vi "加标回收参数设置.vi"() -> ()   [LabVIEW 2016, in "质控单元V4.lvlib"]
panel:
  in  "布尔":bool
  in  "Tab Control 2":enum32{"氨氮", "总磷", "总氮", "高锰酸盐指数", "化学需氧量"}(tab)
  out "氨氮加标回收率":sgl caption="加标回收率" format="%#.2f"
  out "氨氮加标体积":sgl caption="加标体积" format="%#.4f"
  in  "氨氮母液浓度":sgl caption="母液浓度"
  in  "氨氮定容体积":sgl caption="定容体积"
  out "氨氮加标后水样浓度":sgl caption="加标后水样浓度" format="%#.4f"
  out "氨氮加标前水样浓度":sgl caption="加标前水样浓度" format="%#.4f"
  in  "氨氮量程":sgl caption="量程"
  in  "氨氮检出限":sgl caption="检出限"
  out "TP加标回收率":sgl caption="加标回收率" format="%#.2f"
  out "TP加标体积":sgl caption="加标体积" format="%#.4f"
  in  "TP母液浓度":sgl caption="母液浓度"
  in  "TP定容体积":sgl caption="定容体积"
  out "TP加标后水样浓度":sgl caption="加标后水样浓度" format="%#.4f"
  out "TP加标前水样浓度":sgl caption="加标前水样浓度" format="%#.4g"
  in  "TP量程":sgl caption="量程"
  in  "TP检出限":sgl caption="检出限"
  out "TN加标回收率":sgl caption="加标回收率" format="%#.2f"
  out "TN加标体积":sgl caption="加标体积" format="%#.4f"
  in  "TN母液浓度":sgl caption="母液浓度"
  in  "TN定容体积":sgl caption="定容体积"
  out "TN加标后水样浓度":sgl caption="加标后水样浓度" format="%#.4f"
  out "TN加标前水样浓度":sgl caption="加标前水样浓度" format="%#.4f"
  in  "TN量程":sgl caption="量程"
  in  "TN检出限":sgl caption="检出限"
  out "CODMn加标回收率":sgl caption="加标回收率" format="%#.2f"
  out "CODMn加标体积":sgl caption="加标体积" format="%#.4f"
  in  "CODMn母液浓度":sgl caption="母液浓度"
  in  "CODMn定容体积":sgl caption="定容体积"
  out "CODMn加标后水样浓度":sgl caption="加标后水样浓度" format="%#.4f"
  out "CODMn加标前水样浓度":sgl caption="加标前水样浓度" format="%#.4f"
  in  "CODMn量程":sgl caption="量程"
  in  "CODMn检出限":sgl caption="检出限"
  out "CODCr加标回收率":sgl caption="加标回收率" format="%#.2f"
  out "CODCr加标体积":sgl caption="加标体积" format="%#.4f"
  in  "CODCr母液浓度":sgl caption="母液浓度"
  in  "CODCr定容体积":sgl caption="定容体积"
  out "CODCr加标后水样浓度":sgl caption="加标后水样浓度" format="%#.4f"
  out "CODCr加标前水样浓度":sgl caption="加标前水样浓度" format="%#.4f"
  in  "CODCr量程":sgl caption="量程"
  in  "CODCr检出限":sgl caption="检出限"
  # "加标回收参数设置"
  # "加标回收参数"
  # "加标回收参数"
  # "加标回收参数"
  # "加标回收参数"
  # "加标回收参数"
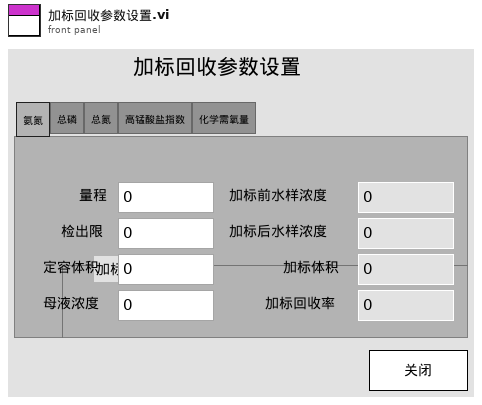
[diagram p1: front panel]
types:
  T1 = cluster{"量程":dbl, "检出限":dbl, "加标前水样浓度":dbl, "加标后水样浓度":dbl, "加标水杯定容体积":dbl, "加标母液浓度":dbl, "加标体积":dbl, "加标回收率":dbl}
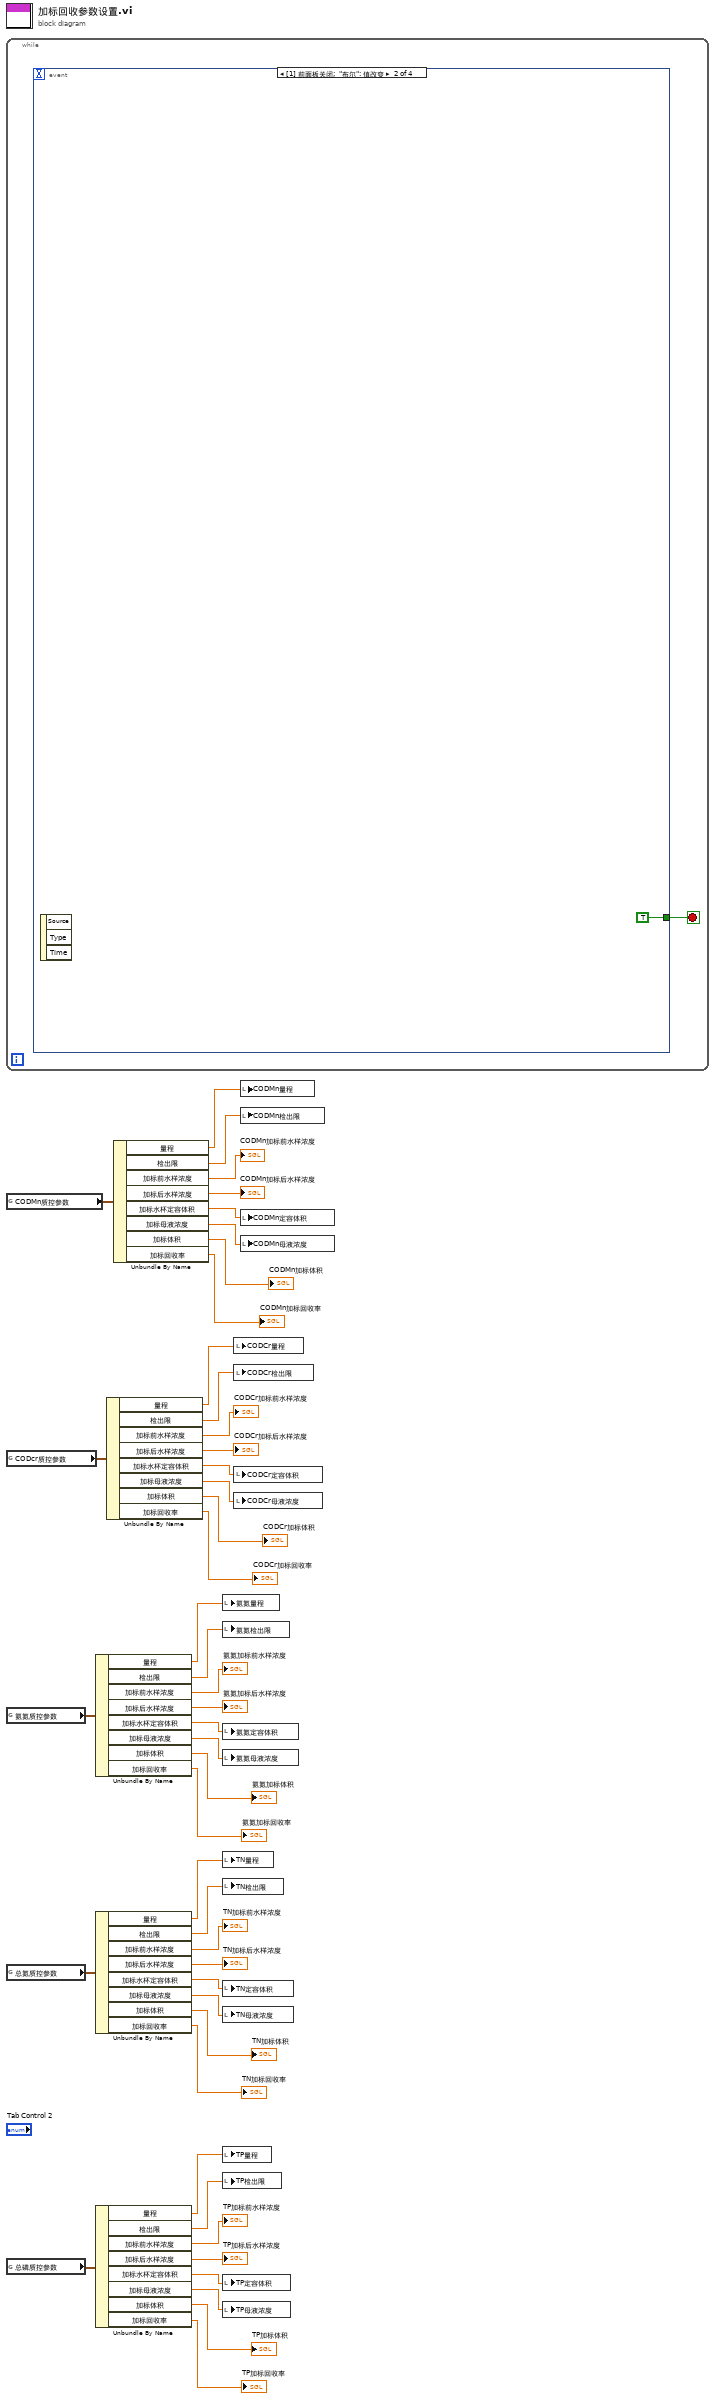
[diagram p0: block diagram]
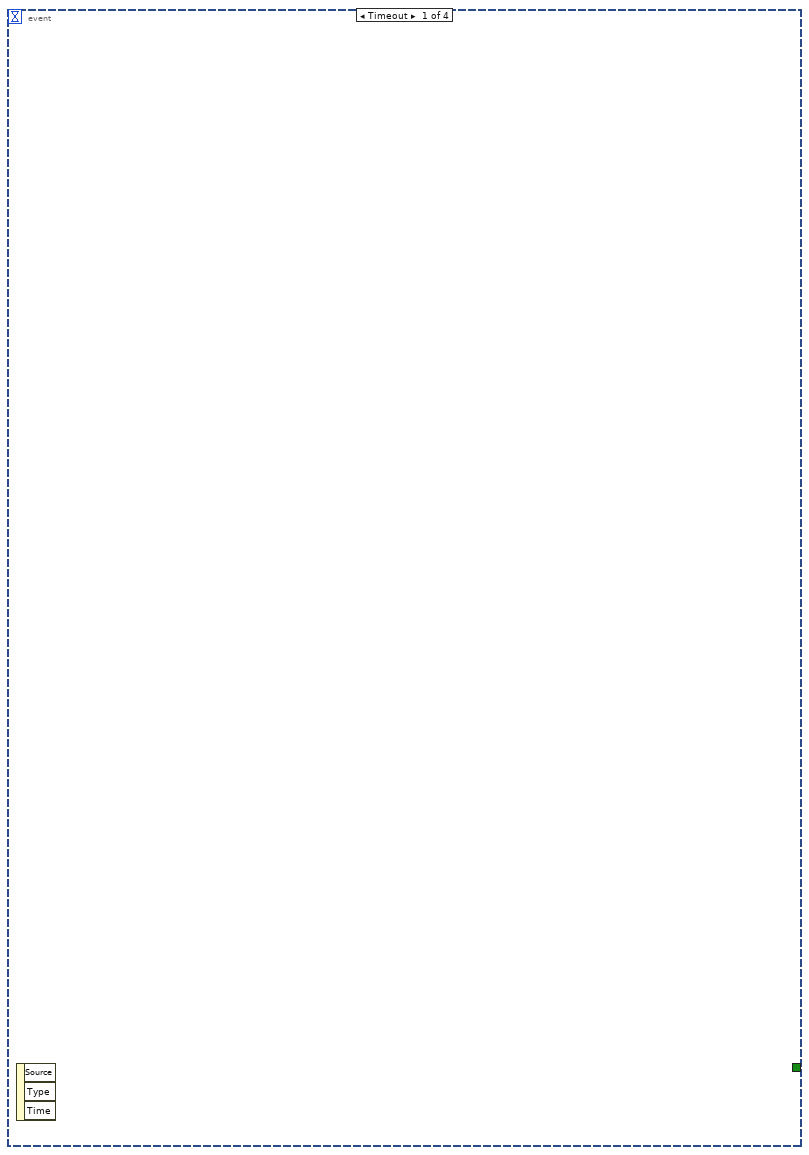
[diagram p2: hidden frame]
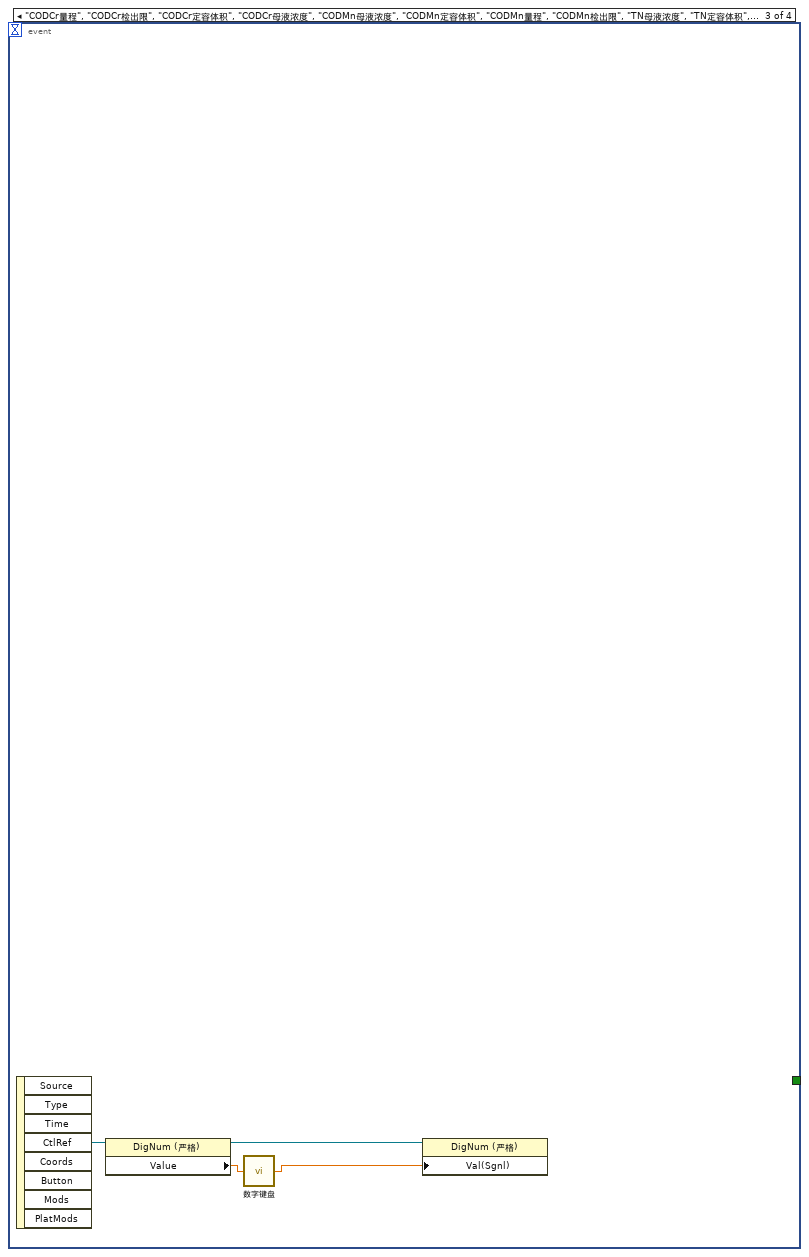
[diagram p3: hidden frame]
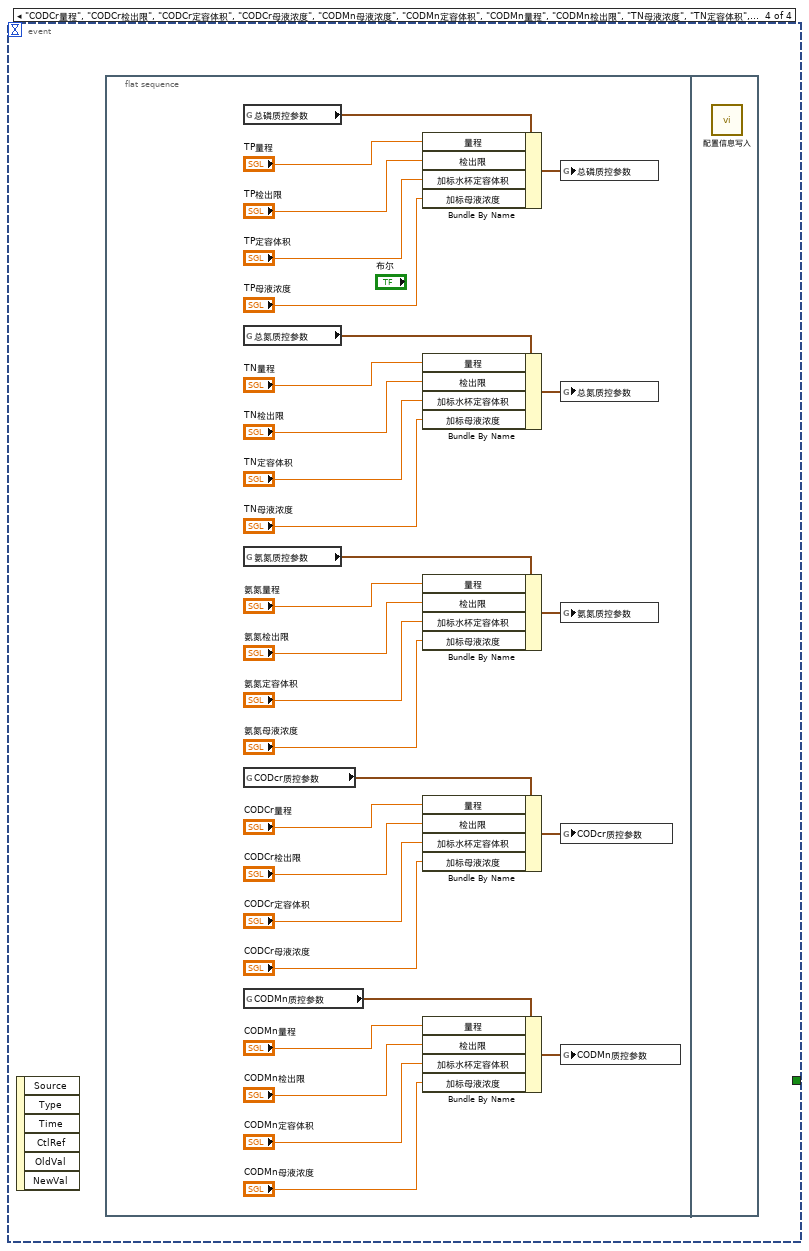
[diagram p4: hidden frame]
diagram:
  n1 = while {
    stop <- w46 stop-if-true
    n2 = event shown="[1] 前面板关闭;  \"布尔\": 值改变" {
      selector: _ -> [_ _ _ _]
      dyn-events: _ -> [_ _ _ _]
      timeout: _ -> [_ _ _ _]
      tunnel: [_ TRUE _ _] -> w46
      event Timeout {
        n3 = event-data() -> ()  [unwired: 1 in, 3 out]
      }
      event Panel Close; "布尔": Value Change {
        n4 = event-data() -> ()  [unwired: 1 in, 3 out]
      }
      event "CODCr量程", "CODCr检出限", "CODCr定容体积", "CODCr母液浓度", "CODMn母液浓度", "CODMn定容体积", "CODMn量程", "CODMn检出限", "TN母液浓度", "TN定容体积", "TN量程", "TN检出限", "TP母液浓度", "TP定容体积", "TP量程", "TP检出限", "氨氮定容体积", "氨氮母液浓度", "氨氮量程", "氨氮检出限": Mouse Down {
        n5 = event-data() -> ("CtlRef"=w51:refnum<vi>)  [unwired: 1 in, 7 out]
        n6 = property class="DigNum (严格)"(reference=w51) -> (reference out=w49:refnum<vi>, "Value"=w50:sgl)  [unwired: 1 in, 1 out]
        n7 = call "数字键盘.vi"("OldNumber"=w50) -> ("NewNumber"=w48:sgl)
        n8 = property class="DigNum (严格)"(reference=w49, "Val(Sgnl)"=w48) -> ()  [unwired: 1 in, 2 out]
      }
      event "CODCr量程", "CODCr检出限", "CODCr定容体积", "CODCr母液浓度", "CODMn母液浓度", "CODMn定容体积", "CODMn量程", "CODMn检出限", "TN母液浓度", "TN定容体积", "TN量程", "TN检出限", "TP母液浓度", "TP定容体积", "TP量程", "TP检出限", "氨氮量程", "氨氮检出限", "氨氮母液浓度", "氨氮定容体积": Value Change {
        n9 = event-data() -> ()  [unwired: 1 in, 6 out]
        n10 = flat-sequence {
          frame #0 {
            n11 = global read "ZK断电保存全局变量.vi" "总磷质控参数"() -> (w57:T1)
            n12 = global read "ZK断电保存全局变量.vi" "总氮质控参数"() -> (w62:T1)
            n13 = global read "ZK断电保存全局变量.vi" "氨氮质控参数"() -> (w69:T1)
            n14 = global read "ZK断电保存全局变量.vi" "CODcr质控参数"() -> (w74:T1)
            n15 = global read "ZK断电保存全局变量.vi" "CODMn质控参数"() -> (w81:T1)
            n16 = Bundle By Name(cluster=w57, "量程"="TP量程", "检出限"="TP检出限", "加标水杯定容体积"="TP定容体积", "加标母液浓度"="TP母液浓度") -> (w56:T1)
            n17 = Bundle By Name(cluster=w62, "量程"="TN量程", "检出限"="TN检出限", "加标水杯定容体积"="TN定容体积", "加标母液浓度"="TN母液浓度") -> (w63:T1)
            n18 = Bundle By Name(cluster=w69, "量程"="氨氮量程", "检出限"="氨氮检出限", "加标水杯定容体积"="氨氮定容体积", "加标母液浓度"="氨氮母液浓度") -> (w68:T1)
            n19 = Bundle By Name(cluster=w74, "量程"="CODCr量程", "检出限"="CODCr检出限", "加标水杯定容体积"="CODCr定容体积", "加标母液浓度"="CODCr母液浓度") -> (w75:T1)
            n20 = Bundle By Name(cluster=w81, "量程"="CODMn量程", "检出限"="CODMn检出限", "加标水杯定容体积"="CODMn定容体积", "加标母液浓度"="CODMn母液浓度") -> (w80:T1)
            n21 = global write "ZK断电保存全局变量.vi" "总磷质控参数"(w56) -> ()
            n22 = global write "ZK断电保存全局变量.vi" "总氮质控参数"(w63) -> ()
            n23 = global write "ZK断电保存全局变量.vi" "氨氮质控参数"(w68) -> ()
            n24 = global write "ZK断电保存全局变量.vi" "CODcr质控参数"(w75) -> ()
            n25 = global write "ZK断电保存全局变量.vi" "CODMn质控参数"(w80) -> ()
          }
          frame #1 {
            n26 = call "配置信息写入.vi"() -> ()  [unwired: 11 in, 1 out]
          }
        }
      }
    }
  }
  n27 = global read "ZK断电保存全局变量.vi" "CODMn质控参数"() -> (w45:T1)
  n28 = global read "ZK断电保存全局变量.vi" "CODcr质控参数"() -> (w36:T1)
  n29 = global read "ZK断电保存全局变量.vi" "氨氮质控参数"() -> (w27:T1)
  n30 = global read "ZK断电保存全局变量.vi" "总氮质控参数"() -> (w18:T1)
  n31 = global read "ZK断电保存全局变量.vi" "总磷质控参数"() -> (w16:T1)
  n32 = Unbundle By Name(w27) -> ("量程"=w22:dbl, "检出限"=w21:dbl, "加标前水样浓度"=→"氨氮加标前水样浓度":dbl, "加标后水样浓度"=→"氨氮加标后水样浓度":dbl, "加标水杯定容体积"=w20:dbl, "加标母液浓度"=w19:dbl, "加标体积"=→"氨氮加标体积":dbl, "加标回收率"=→"氨氮加标回收率":dbl)
  n33 = Unbundle By Name(w18) -> ("量程"=w4:dbl, "检出限"=w3:dbl, "加标前水样浓度"=→"TN加标前水样浓度":dbl, "加标后水样浓度"=→"TN加标后水样浓度":dbl, "加标水杯定容体积"=w2:dbl, "加标母液浓度"=w1:dbl, "加标体积"=→"TN加标体积":dbl, "加标回收率"=→"TN加标回收率":dbl)
  n34 = Unbundle By Name(w16) -> ("量程"=w8:dbl, "检出限"=w7:dbl, "加标前水样浓度"=→"TP加标前水样浓度":dbl, "加标后水样浓度"=→"TP加标后水样浓度":dbl, "加标水杯定容体积"=w6:dbl, "加标母液浓度"=w5:dbl, "加标体积"=→"TP加标体积":dbl, "加标回收率"=→"TP加标回收率":dbl)
  n35 = Unbundle By Name(w36) -> ("量程"=w31:dbl, "检出限"=w30:dbl, "加标前水样浓度"=→"CODCr加标前水样浓度":dbl, "加标后水样浓度"=→"CODCr加标后水样浓度":dbl, "加标水杯定容体积"=w29:dbl, "加标母液浓度"=w28:dbl, "加标体积"=→"CODCr加标体积":dbl, "加标回收率"=→"CODCr加标回收率":dbl)
  n36 = Unbundle By Name(w45) -> ("量程"=w40:dbl, "检出限"=w39:dbl, "加标前水样浓度"=→"CODMn加标前水样浓度":dbl, "加标后水样浓度"=→"CODMn加标后水样浓度":dbl, "加标水杯定容体积"=w38:dbl, "加标母液浓度"=w37:dbl, "加标体积"=→"CODMn加标体积":dbl, "加标回收率"=→"CODMn加标回收率":dbl)
  n37 = local write "氨氮量程"(w22) -> ()
  n38 = local write "氨氮检出限"(w21) -> ()
  n39 = local write "氨氮定容体积"(w20) -> ()
  n40 = local write "氨氮母液浓度"(w19) -> ()
  n41 = local write "TN量程"(w4) -> ()
  n42 = local write "TN检出限"(w3) -> ()
  n43 = local write "TN定容体积"(w2) -> ()
  n44 = local write "TN母液浓度"(w1) -> ()
  n45 = local write "TP量程"(w8) -> ()
  n46 = local write "TP检出限"(w7) -> ()
  n47 = local write "TP定容体积"(w6) -> ()
  n48 = local write "TP母液浓度"(w5) -> ()
  n49 = local write "CODCr量程"(w31) -> ()
  n50 = local write "CODCr检出限"(w30) -> ()
  n51 = local write "CODCr定容体积"(w29) -> ()
  n52 = local write "CODCr母液浓度"(w28) -> ()
  n53 = local write "CODMn量程"(w40) -> ()
  n54 = local write "CODMn检出限"(w39) -> ()
  n55 = local write "CODMn定容体积"(w38) -> ()
  n56 = local write "CODMn母液浓度"(w37) -> ()
